vi "read wait ms.vi"(8 "error in (no error)":errorcluster caption="entrée d'erreur (pas d'erreur)", 11 "DelayLineLS4 en entrée":refnum<class "DelayLineLS4.lvclass">) -> (0 "error out":errorcluster caption="sortie d'erreur", 2 "wait ms":i32 min=0 max=1000, 3 "DelayLineLS4 en sortie":refnum<class "DelayLineLS4.lvclass">)   [LabVIEW 2015, in "DelayLineLS4.lvclass"]
uses:
  DelayLineLS4.lvclass
  DelayLineLS4.lvclass/DelayLineLS4.ctl
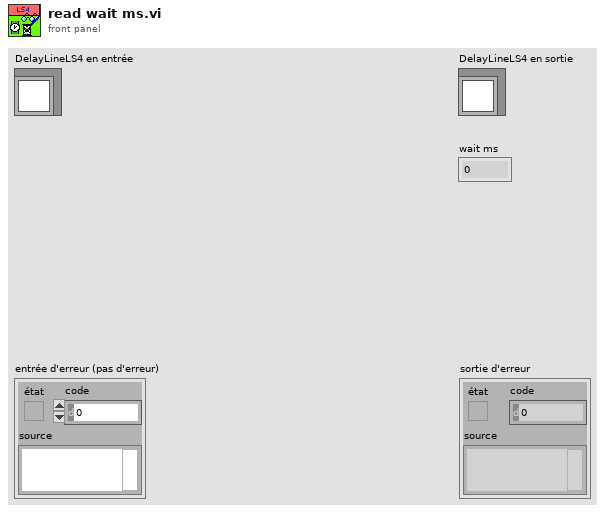
[diagram p1: front panel]
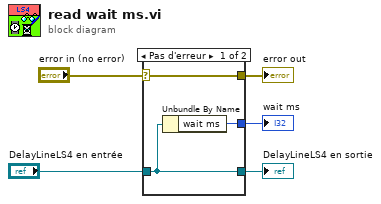
[diagram p0: block diagram]
diagram:
  n1 = case shown="Pas d'erreur" "error in (no error)" {
    selector: "error in (no error)" -> [w8 w9]
    tunnel: [w8 w9] -> w4
    tunnel: [w7 w10] -> w2
    tunnel: "DelayLineLS4 en entrée" -> [w7 w10]
    tunnel: [w6 _] -> w1
    frame No Error {
      n2 = Unbundle By Name(w7) -> ("wait ms"=w6:i32)
    }
    frame Error {
    }
  }
  "error out" <- w4
  "DelayLineLS4 en sortie" <- w2
  "wait ms" <- w1
